vi "2DMain.vi"() -> (0 "Timestep":dbl=0.1 format="%#_13g", 1 "Heading":dbl[](array[numeric]), 2 "Right":cluster{"Distance":dbl[], "Velocity":dbl[]}, 3 "Left":cluster{"Distance":dbl[], "Velocity":dbl[]})   [LabVIEW 2016]
panel:
  out "x-y":dbl
  out "XY Graph":cluster{"X":dbl, "Y":dbl}[](graph)
  in  "TrackWidth":dbl=35.0 format="%#_13g"
  out "Distance":cluster{"Array Out":dbl[], "Array Out":dbl[]}[](graph)=[{"Array Out"=[0.0, 0.1, 0.2, 0.30000000000000004, 0.4, 0.5, 0.6, 0.7, 0.7999999999999999, 0.8999999999999999, 0.9999999999999999, 1.0999999999999999, 1.1999999999999997, 1.2999999999999998, 1.4, 1.5, 1.6, 1.7000000000000002, 1.8000000000000003, 1.9000000000000004, 2.0000000000000004, 2.1000000000000005, 2.2000000000000006, 2.3000000000000007, 2.400000000000001, 2.500000000000001, 2.600000000000001, 2.700000000000001, 2.800000000000001, 2.9000000000000012, 3.0000000000000013, 3.1000000000000014, 3.2000000000000015, 3.3000000000000016, 3.4000000000000017, 3.5000000000000018, 3.600000000000002, 3.700000000000002, 3.800000000000002, 3.900000000000002, 4.000000000000002, 4.100000000000001, 4.200000000000001, 4.300000000000001, 4.4, 4.5, 4.6, 4.699999999999999, 4.799999999999999, 4.899999999999999, 4.999999999999998, 5.099999999999998, 5.1999999999999975, 5.299999999999997, 5.399999999999997, 5.4999999999999964, 5.599999999999996, 5.699999999999996, 5.799999999999995, 5.899999999999995, 5.999999999999995, 6.099999999999994, 6.199999999999994, 6.299999999999994, 6.399999999999993, 6.499999999999993, 6.5999999999999925, 6.699999999999992, 6.799999999999992, 6.8999999999999915, 6.999999999999991, 7.099999999999991, 7.19999999999999, 7.29999999999999, 7.39999999999999, 7.499999999999989], "Array Out"=[0.20069481389041308, 1.2735479131566998, 2.860563643560315, 4.677475723799337, 6.602913279626835, 8.567527988927633, 10.53108018964165, 12.465647282368936, 14.34875346161623, 16.16309622777655, 17.898491074990865, 19.549502803192667, 21.10424300305833, 22.544365069194978, 23.85409275892922, 25.03102772342022, 26.085867448969292, 27.022262629224457, 27.841084013292193, 28.562821763985134, 29.232471840215105, 29.873513699283382, 30.508866157063213, 31.172262554607624, 31.908022069990984, 32.78038389904512, 33.86754429730758, 35.198256581265305, 36.75501986546203, 38.50844318386972, 40.44050862786903, 42.54224982283954, 44.78915116071239, 47.14602178312011, 49.584921471, 52.097800881345535, 54.690898184409775, 57.359640143421814, 60.0931923583142, 62.893846806981905, 65.79097479873057, 68.83230748850526, 72.05193120455107, 75.47740260353666, 79.15300666582458, 83.15137230577258, 87.55638168234262, 92.42537513448103, 97.79978506553392, 103.7283633518359, 110.27176098442025, 117.47770658119887, 125.34310783591802, 133.82920697375735, 142.8898773894898, 152.48590627079324, 162.58103064590355, 173.12865405386947, 184.07735731984107, 195.38107047923268, 207.00308349309873, 218.91193352626502, 231.07343083234156, 243.45198855767703, 256.01410216111213, 268.72824012658504, 281.5595738656088, 294.46074577221134, 307.3634720865251, 320.16447276700615, 332.6976768600146, 344.6827382996951, 355.6340519955303, 364.70338314474, 370.3292731264785, 371.34805932997506]}, {"Array Out"=[0.0, 0.1, 0.2, 0.30000000000000004, 0.4, 0.5, 0.6, 0.7, 0.7999999999999999, 0.8999999999999999, 0.9999999999999999, 1.0999999999999999, 1.1999999999999997, 1.2999999999999998, 1.4, 1.5, 1.6, 1.7000000000000002, 1.8000000000000003, 1.9000000000000004, 2.0000000000000004, 2.1000000000000005, 2.2000000000000006, 2.3000000000000007, 2.400000000000001, 2.500000000000001, 2.600000000000001, 2.700000000000001, 2.800000000000001, 2.9000000000000012, 3.0000000000000013, 3.1000000000000014, 3.2000000000000015, 3.3000000000000016, 3.4000000000000017, 3.5000000000000018, 3.600000000000002, 3.700000000000002, 3.800000000000002, 3.900000000000002, 4.000000000000002, 4.100000000000001, 4.200000000000001, 4.300000000000001, 4.4, 4.5, 4.6, 4.699999999999999, 4.799999999999999, 4.899999999999999, 4.999999999999998, 5.099999999999998, 5.1999999999999975, 5.299999999999997, 5.399999999999997, 5.4999999999999964, 5.599999999999996, 5.699999999999996, 5.799999999999995, 5.899999999999995, 5.999999999999995, 6.099999999999994, 6.199999999999994, 6.299999999999994, 6.399999999999993, 6.499999999999993, 6.5999999999999925, 6.699999999999992, 6.799999999999992, 6.8999999999999915, 6.999999999999991, 7.099999999999991, 7.19999999999999, 7.29999999999999, 7.39999999999999, 7.499999999999989], "Array Out"=[0.2117191306056528, 1.3507882424896287, 3.071429044529173, 5.09397779407175, 7.301900538479339, 9.628251136963636, 12.034681936226827, 14.503404614724442, 17.02963034745262, 19.613660791751258, 22.25469422033156, 24.951328686393314, 27.711896764961377, 30.553446132360143, 33.49237898778358, 36.53443998973933, 39.67669409791384, 42.929661075996734, 46.31492189548162, 49.84503113661403, 53.50368108524415, 57.25169961687586, 61.07026124095799, 64.95859991137544, 68.90728696067245, 72.88101782758629, 76.83587578292126, 80.76784216096199, 84.70462040360079, 88.6778427280159, 92.70471482207125, 96.79005649072815, 100.94903919796458, 105.2061488333065, 109.58233928983002, 114.08475664593064, 118.71116835031577, 123.47309491255056, 128.3941338888642, 133.49475313859787, 138.77995304825606, 144.24552491424538, 149.90687713291584, 155.7961174670011, 161.94399225424323, 168.36714991065222, 175.07505744482475, 182.09686270564254, 189.47668975565475, 197.25604197786453, 205.4591611195571, 214.09006503805574, 223.14687047737073, 232.6258465985691, 242.52047336593304, 252.81806385202069, 263.4961069829394, 274.5251855181033, 285.87506411948084, 297.5184169240899, 309.4300792332615, 321.5837023958519, 333.95091437242615, 346.5036236619891, 359.2151167805168, 372.0578239392519, 384.9981906850866, 397.9905683314788, 410.969322166184, 423.8337224292351, 436.4191499472047, 448.4455434819155, 459.42763327185486, 468.5178463185088, 474.1549337579138, 475.1756544408442]}]
  in  "Path":i32=4
  in  "Timestep":dbl=0.1 format="%#_13g"
  out "Pos":cluster{"Array Out":dbl[], "Array Out":dbl[]}[](graph)=[{"Array Out"=[0.0, 0.0, 100.0, 100.0], "Array Out"=[0.0, -50.0, -50.0, 300.0]}, {"Array Out"=[0.0, 0.23102521238156823, 0.46462967685251366, 0.7037123278438489, 0.9517380195633947, 1.212752350834045, 1.4907899822064303, 1.78783247902104, 2.1065958337168587, 2.451695954720305, 2.8296673375725714, 3.247334487022741, 3.706724316460749, 4.211245916492695, 4.768155922064141, 5.388574268428332, 6.084254547225372, 6.857720318418225, 7.713840686939641, 8.664326744157881, 9.727605490171953, 10.922685952772534, 12.250880804587691, 13.716104501567363, 15.332115456656412, 17.121095424852708, 19.101090310427278, 21.251474961621344, 23.547168687359076, 25.970948218634163, 28.514853498873496, 31.173537193331367, 33.9260087077582, 36.751125048786044, 39.63255921600619, 42.55890760852029, 45.520822161399416, 48.504522369702826, 51.495479207803186, 54.47917940610018, 57.44109393904035, 60.367442301904724, 63.248876430343955, 66.07399272417004, 68.82646418372462, 71.48514781641364, 74.02905302884325, 76.4528324873993, 78.74852613667896, 80.89891070878437, 82.87890551366146, 84.66788540053744, 86.28389627482022, 87.7491198925626, 89.07731466758672, 90.27239505652396, 91.3356737325474, 92.28615972405139, 93.14228003158937, 93.91574574676325, 94.61142597452503, 95.23184427472546, 95.78875423897482, 96.29327580240847, 96.75266559972492, 97.17033272118528, 97.54830407983745, 97.89340418031219, 98.21216751811241, 98.50921000167841, 98.78724762354712, 99.04826194932421, 99.29628764016333, 99.53537029562708, 99.76897477062725, 100.0], "Array Out"=[0.0, -1.827838650398022, -3.65375518167116, -5.475589233211732, -7.290758689387357, -9.096248608842847, -10.889052113698222, -12.66769215834793, -14.430144140207465, -16.1729671902586, -17.89128995963179, -19.58002374541511, -21.237652967227923, -22.86162855610636, -24.446528413729688, -25.98404181136415, -27.46536978319958, -28.888565190622653, -30.249889534074487, -31.540434698254117, -32.74617284968212, -33.85245754230255, -34.85753541640947, -35.75725126468736, -36.5393970689817, -37.18439938874207, -37.674159806617034, -38.017116888370275, -38.221986911053236, -38.28800121444147, -38.20416326811608, -37.95711557222517, -37.55408282907005, -36.998920290461676, -36.28324747689388, -35.386328053162075, -34.28454694169509, -32.97910678617733, -31.4655419732727, -29.722082598161755, -27.70960719661141, -25.385571609721282, -22.745546720347345, -19.776058061619167, -16.436505113053137, -12.659603644587932, -8.375157173488198, -3.5804811976422233, 1.737307919479062, 7.6291113212396535, 14.178887353926195, 21.456950034459567, 29.39106322953373, 37.89510823042944, 46.915601776628804, 56.43664528918128, 66.45254738703716, 76.89163453916119, 87.68459791049352, 98.78739611010738, 110.18168332188421, 121.85794172593427, 133.7721115823067, 145.88252235746378, 158.16198204859364, 170.59771431455354, 183.18212283436563, 195.8896453923813, 208.6958071543085, 221.58331952589336, 234.54200992609125, 247.5644566117797, 260.6355487239612, 273.7401345254334, 286.86523733837987, 300.0]}, {"Array Out"=[17.361870832049785, 17.589538187103535, 17.815857798056786, 18.042596925983897, 18.271683704856557, 18.506023628599557, 18.751734565427235, 19.008441820362023, 19.27328878543838, 19.543098566247437, 19.817797247594193, 20.111683112592367, 20.418804411748653, 20.721624708223516, 20.996721817172322, 21.228727153803682, 21.46022876404934, 21.67174743661132, 21.804621956763874, 21.789771454866482, 21.61567635194309, 21.482648386286343, 21.408110180164382, 21.340039996418675, 21.267603745103752, 21.32315569414887, 21.85726926108888, 22.807010778665354, 24.023623763946112, 25.394524261530325, 26.89571010192149, 28.638122467704868, 30.55162586861914, 32.53275092193286, 34.50431716952587, 36.4576564551441, 38.50617093018464, 40.6028384312195, 42.66652607308066, 44.644190057731024, 46.55766616939471, 48.54539998819105, 50.5701354162769, 52.569682235036375, 54.516392831550185, 56.43771311124984, 58.41118035051687, 60.38605479951565, 62.30924164299841, 64.14759026827126, 65.88476780432264, 67.51996237076557, 69.03800784797089, 70.43579160738425, 71.71356515707643, 72.87017958701705, 73.90776528104465, 74.8409562086548, 75.68459052136886, 76.44827251516784, 77.13607793295802, 77.75093135418209, 78.303920722879, 78.80550946903678, 79.26252745611387, 79.67822071408006, 80.05475373216495, 80.3988230045449, 80.71681410433365, 81.0132366438934, 81.290761777104, 81.55141158543043, 81.79919935740034, 82.03814145672865, 82.27168110629135, 82.5027063356641], "Array Out"=[2.194411358706214, 0.39297816023924836, -1.376721434461866, -3.1063950891235277, -4.786865429183404, -6.414314882292096, -8.006381113569976, -9.553111301648318, -11.030930539782403, -12.413451693458054, -13.689690007205483, -14.90629445979662, -16.04569968462976, -17.0601294262637, -17.897967580376175, -18.544985650268515, -19.108970027110566, -19.57220321067363, -19.872034109856507, -19.96577698641954, -19.903907816382578, -19.897630656856172, -19.94461651489742, -20.005247977157666, -20.076712634852967, -20.196383333498815, -20.392566199778283, -20.58638803608492, -20.7284740974416, -20.797497064426906, -20.77922784039909, -20.641756142831962, -20.38249174219275, -20.014947853899738, -19.551507175517234, -18.984354563260755, -18.2519343004436, -17.36458178743611, -16.355956057541146, -15.247173806826824, -14.005556701122641, -12.482497730495313, -10.683228274119283, -8.645757157642022, -6.363181039259199, -3.725136184586079, -0.48009206903298374, 3.3555590796430605, 7.737301697462016, 12.693029122630946, 18.356121309072584, 24.949618894374467, 32.36248248111438, 40.444355901732294, 49.095097804671475, 58.28404799375175, 68.03937031541905, 78.2754243737801, 88.90077099222853, 99.8538757880656, 111.11023640388856, 122.6750607285158, 134.50053241837068, 146.53676135767063, 158.74940669686964, 171.123088020486, 183.65719781102453, 196.32511006889226, 209.09905512638045, 221.95870767658198, 234.8926992832377, 247.89646164714847, 260.95476906353554, 274.05155539695886, 287.17299442439236, 300.3077570860125]}, {"Array Out"=[-17.361870832049785, -17.1274877623404, -16.88659844435176, -16.6351722702962, -16.36820766572977, -16.080518926931468, -15.770154601014376, -15.432776862319942, -15.06009711800466, -14.639706656806828, -14.158462572449052, -13.617014138546885, -13.005355778827154, -12.299132875238124, -11.460409973044035, -10.45157861694702, -9.291719669598594, -7.9563067997748655, -6.376940582884591, -4.461117966550717, -2.16046537159918, 0.36272351925873103, 3.093651429011002, 6.092169006716055, 9.396627168209074, 12.919035155556548, 16.344911359765675, 19.695939144577338, 23.070713610772042, 26.547372175738, 30.133996895825504, 33.708951918957865, 37.30039154689726, 40.96949917563923, 44.76080126248652, 48.66015876189649, 52.53547339261419, 56.40620630818615, 60.32443234252571, 64.31416875446934, 68.324521708686, 72.1894846156184, 75.92761744441101, 79.57830321330371, 83.13653553589907, 86.53258252157744, 89.64692570716963, 92.51961017528296, 95.18781063035951, 97.65023114929748, 99.8730432230003, 101.81580843030932, 103.52978470166956, 105.06244817774096, 106.44106417809701, 107.67461052603088, 108.76358218405016, 109.73136323944797, 110.59996954180987, 111.38321897835866, 112.08677401609205, 112.71275719526884, 113.27358775507065, 113.78104213578017, 114.24280374333597, 114.6624447282905, 115.04185442750995, 115.38798535607948, 115.70752093189117, 116.00518335946342, 116.28373346999024, 116.545112313218, 116.79337592292632, 117.0325991345255, 117.26626843496315, 117.4972936643359], "Array Out"=[-2.19441135870622, -4.048655461035298, -5.930788928880457, -7.8447833772999385, -9.794651949591312, -11.778182335393597, -13.77172311382647, -15.782273015047544, -17.829357740632524, -19.932482687059153, -22.092889912058098, -24.2537530310336, -26.42960624982609, -28.663127685949025, -30.995089247083204, -33.423097972459786, -35.821769539288596, -38.20492717057168, -40.627744958292475, -43.11509241008869, -45.588437882981665, -47.80728442774894, -49.77045431792152, -51.50925455221706, -53.00208150311043, -54.17241544398533, -54.95575341345578, -55.44784574065564, -55.715499724664866, -55.77850536445604, -55.62909869583308, -55.272475001618375, -54.72567391594734, -53.98289272702361, -53.014987778270516, -51.7883015430634, -50.31715958294657, -48.59363178491856, -46.57512788900425, -44.19699138949669, -41.41365769210018, -38.28864548894725, -34.807865166575404, -30.90635896559631, -26.50982918684707, -21.594071104589787, -16.270222277943414, -10.516521474927508, -4.26268585850389, 2.5651935198483606, 10.001653398779801, 17.964281174544666, 26.419643977953086, 35.34586055912659, 44.73610574858614, 54.58924258461081, 64.86572445865527, 75.50784470454228, 86.46842482875851, 97.72091643214917, 109.25313023987987, 121.04082272335275, 133.04369074624276, 145.22828335725694, 157.57455740031764, 170.0723406086211, 182.70704785770673, 195.45418071587036, 208.29255918223654, 221.20793137520474, 234.1913205689448, 247.2324515764109, 260.3163283843869, 273.42871365390795, 286.5574802523674, 299.6922429139875]}]
  in  "B":dbl=0.3 format="%#_13g"
  in  "A":dbl=0.1 format="%#_13g"
  out "Vel":cluster{"Array Out":dbl[], "Array Out":dbl[]}[](graph)=[{"Array Out"=[0.0, 0.1, 0.2, 0.30000000000000004, 0.4, 0.5, 0.6, 0.7, 0.7999999999999999, 0.8999999999999999, 0.9999999999999999, 1.0999999999999999, 1.1999999999999997, 1.2999999999999998, 1.4, 1.5, 1.6, 1.7000000000000002, 1.8000000000000003, 1.9000000000000004, 2.0000000000000004, 2.1000000000000005, 2.2000000000000006, 2.3000000000000007, 2.400000000000001, 2.500000000000001, 2.600000000000001, 2.700000000000001, 2.800000000000001, 2.9000000000000012, 3.0000000000000013, 3.1000000000000014, 3.2000000000000015, 3.3000000000000016, 3.4000000000000017, 3.5000000000000018, 3.600000000000002, 3.700000000000002, 3.800000000000002, 3.900000000000002, 4.000000000000002, 4.100000000000001, 4.200000000000001, 4.300000000000001, 4.4, 4.5, 4.6, 4.699999999999999, 4.799999999999999, 4.899999999999999, 4.999999999999998, 5.099999999999998, 5.1999999999999975, 5.299999999999997, 5.399999999999997, 5.4999999999999964, 5.599999999999996, 5.699999999999996, 5.799999999999995, 5.899999999999995, 5.999999999999995, 6.099999999999994, 6.199999999999994, 6.299999999999994, 6.399999999999993, 6.499999999999993, 6.5999999999999925, 6.699999999999992, 6.799999999999992, 6.8999999999999915, 6.999999999999991, 7.099999999999991, 7.19999999999999, 7.29999999999999, 7.39999999999999, 7.499999999999989], "Array Out"=[0.0, 12.372404710634475, 16.867961965733866, 19.38524707805461, 20.774503850816224, 21.516879350956227, 21.88575500916673, 22.03750338231366, 22.059246850404637, 21.99898976068586, 21.884595775786014, 21.735465316179884, 21.567838010185906, 21.39086636490795, 21.21078614022004, 21.036380652168358, 20.88260524384004, 20.769595460208766, 20.71554064077986, 20.741238149163674, 20.87312553452902, 21.139138505559412, 21.558196840969877, 22.146332757903, 22.920286281934025, 23.884942406325237, 25.00730511015754, 26.201615050928723, 27.406330399265517, 28.598837650755197, 29.777101396449172, 30.93184938112929, 32.03182897947415, 33.07141598551832, 34.072723255157534, 35.07007214021115, 36.090131871364406, 37.14130978100209, 38.25204996283135, 39.474815512695244, 40.87180169401338, 42.49139031558557, 44.35340950392369, 46.50833340172636, 49.038853444879535, 52.025168577610394, 55.492180787293826, 59.38244543220561, 63.69363759700799, 68.4639215492525, 73.68404574590186, 79.19222262081749, 84.65051888907514, 89.87067775320472, 94.81830414769881, 99.51459563457516, 103.93164470775784, 107.95370522362096, 111.55450817401655, 114.78566877837973, 117.71476648458234, 120.36550738532917, 122.69738889857928, 124.70620834771844, 126.41578314831844, 127.8388568944075, 128.93413980879347, 129.57559553511445, 129.5699618807708, 128.5889586621701, 126.03622897115463, 120.82507088621556, 111.00713371098406, 93.14849572458364, 61.185206037126065, 0.0]}, {"Array Out"=[0.0, 0.1, 0.2, 0.30000000000000004, 0.4, 0.5, 0.6, 0.7, 0.7999999999999999, 0.8999999999999999, 0.9999999999999999, 1.0999999999999999, 1.1999999999999997, 1.2999999999999998, 1.4, 1.5, 1.6, 1.7000000000000002, 1.8000000000000003, 1.9000000000000004, 2.0000000000000004, 2.1000000000000005, 2.2000000000000006, 2.3000000000000007, 2.400000000000001, 2.500000000000001, 2.600000000000001, 2.700000000000001, 2.800000000000001, 2.9000000000000012, 3.0000000000000013, 3.1000000000000014, 3.2000000000000015, 3.3000000000000016, 3.4000000000000017, 3.5000000000000018, 3.600000000000002, 3.700000000000002, 3.800000000000002, 3.900000000000002, 4.000000000000002, 4.100000000000001, 4.200000000000001, 4.300000000000001, 4.4, 4.5, 4.6, 4.699999999999999, 4.799999999999999, 4.899999999999999, 4.999999999999998, 5.099999999999998, 5.1999999999999975, 5.299999999999997, 5.399999999999997, 5.4999999999999964, 5.599999999999996, 5.699999999999996, 5.799999999999995, 5.899999999999995, 5.999999999999995, 6.099999999999994, 6.199999999999994, 6.299999999999994, 6.399999999999993, 6.499999999999993, 6.5999999999999925, 6.699999999999992, 6.799999999999992, 6.8999999999999915, 6.999999999999991, 7.099999999999991, 7.19999999999999, 7.29999999999999, 7.39999999999999, 7.499999999999989], "Array Out"=[0.0, 12.703147836339168, 17.53155536768189, 20.40907881530594, 22.18505434364899, 23.326068474553402, 24.091707667195205, 24.69294881245726, 25.259857792832722, 25.841163979902532, 26.4173129454754, 26.95158995301414, 27.574395206173122, 28.384913936377217, 29.378911092243946, 30.435413020053282, 31.40309694488795, 32.48744569086545, 33.82513897662405, 35.32764757173127, 36.670825204395705, 37.50804852849331, 38.178092579533704, 38.89327859829959, 39.54911325231494, 39.83149135026113, 39.54877336147123, 39.264892523952234, 39.30963922516325, 39.70324513372229, 40.270719704855075, 40.8262016901782, 41.54497365384626, 42.53286612862268, 43.75013995217846, 45.0380014540742, 46.24289559756238, 47.57511841878443, 49.172224461387486, 50.99832231448317, 52.87164126470022, 54.6271072062081, 56.55424186982691, 58.83705843471155, 61.45194443644167, 64.22765105405034, 67.02691073189621, 70.13915806871688, 73.72477264230297, 77.75137436280403, 82.03086323906707, 86.3123211824826, 90.57408714092081, 94.79965661273292, 98.96585368004982, 103.01453470890381, 106.83143664959356, 110.34230654784649, 113.5440492688524, 116.47421245939738, 119.16026917009916, 121.58444941050175, 123.71932294331766, 125.57097741068446, 127.1593247877209, 128.4813105500948, 129.477862536004, 130.02924405597452, 129.94782002362786, 128.90470593182337, 126.29737203214363, 121.03145701777747, 111.160411979395, 93.25228246100522, 61.243240975823106, 0.0]}, {"Array Out"=[0.0, 0.1, 0.2, 0.30000000000000004, 0.4, 0.5, 0.6, 0.7, 0.7999999999999999, 0.8999999999999999, 0.9999999999999999, 1.0999999999999999, 1.1999999999999997, 1.2999999999999998, 1.4, 1.5, 1.6, 1.7000000000000002, 1.8000000000000003, 1.9000000000000004, 2.0000000000000004, 2.1000000000000005, 2.2000000000000006, 2.3000000000000007, 2.400000000000001, 2.500000000000001, 2.600000000000001, 2.700000000000001, 2.800000000000001, 2.9000000000000012, 3.0000000000000013, 3.1000000000000014, 3.2000000000000015, 3.3000000000000016, 3.4000000000000017, 3.5000000000000018, 3.600000000000002, 3.700000000000002, 3.800000000000002, 3.900000000000002, 4.000000000000002, 4.100000000000001, 4.200000000000001, 4.300000000000001, 4.4, 4.5, 4.6, 4.699999999999999, 4.799999999999999, 4.899999999999999, 4.999999999999998, 5.099999999999998, 5.1999999999999975, 5.299999999999997, 5.399999999999997, 5.4999999999999964, 5.599999999999996, 5.699999999999996, 5.799999999999995, 5.899999999999995, 5.999999999999995, 6.099999999999994, 6.199999999999994, 6.299999999999994, 6.399999999999993, 6.499999999999993, 6.5999999999999925, 6.699999999999992, 6.799999999999992, 6.8999999999999915, 6.999999999999991, 7.099999999999991, 7.19999999999999, 7.29999999999999, 7.39999999999999, 7.499999999999989], "Array Out"=[0.0, 12.041688833424784, 16.204430622278075, 18.36153250167981, 19.36416418534402, 19.70806410659394, 19.68046194632811, 19.383220150934577, 18.86068301357076, 18.160418549620026, 17.358208757568306, 16.530437252965662, 15.580745922677252, 14.430991048264993, 13.102613852461802, 11.742214925942376, 10.544624313228791, 9.369671354086913, 8.16040108573351, 7.118007347043244, 6.671834567670051, 6.373658956074809, 6.2960411521273825, 6.563323902205564, 7.254447091715027, 8.564458653936002, 10.829428035789238, 13.34745309865494, 15.623496607054237, 17.56435752493153, 19.324472397681014, 21.061679524302914, 22.53328120333792, 23.619275934716914, 24.40185240225773, 25.107295729045656, 25.941729302291556, 26.711625245642534, 27.336287255860423, 27.95635862445902, 28.87754516636604, 30.3611402149965, 32.15785536012971, 34.18486130723312, 36.630983350072995, 39.827449029750035, 43.96115892780746, 48.62847785322212, 53.664536787609045, 59.17797085951554, 65.33827695244722, 72.07277928575733, 78.72734171124067, 84.941929152429, 90.67088994940376, 96.0147359939041, 101.03189895318627, 105.56513069996929, 109.56498272489092, 113.09713435876397, 116.26926940354987, 119.14656885900025, 121.67545715042685, 123.84144090388503, 125.6722427541605, 127.19640428557923, 128.3904180318958, 129.12194792826241, 129.19210465120622, 128.27321232573897, 125.77508687469972, 120.61868575596885, 110.85385648225208, 93.04471006513418, 61.127172209794075, 0.0]}]
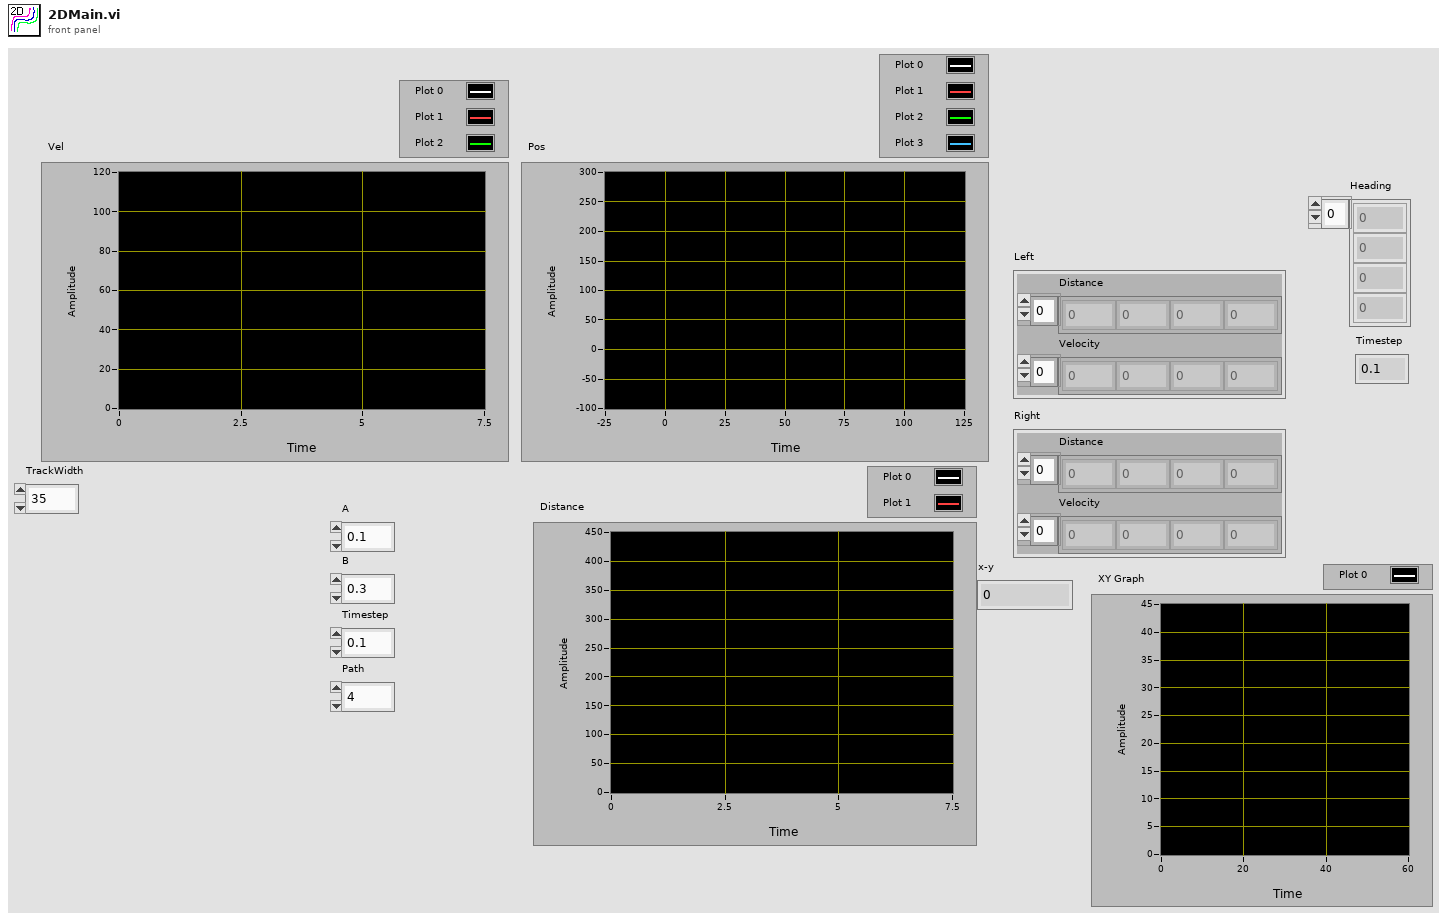
[diagram p1: front panel]
types:
  T1 = cluster{"transposed array":dbl[], "transposed array":dbl[]}
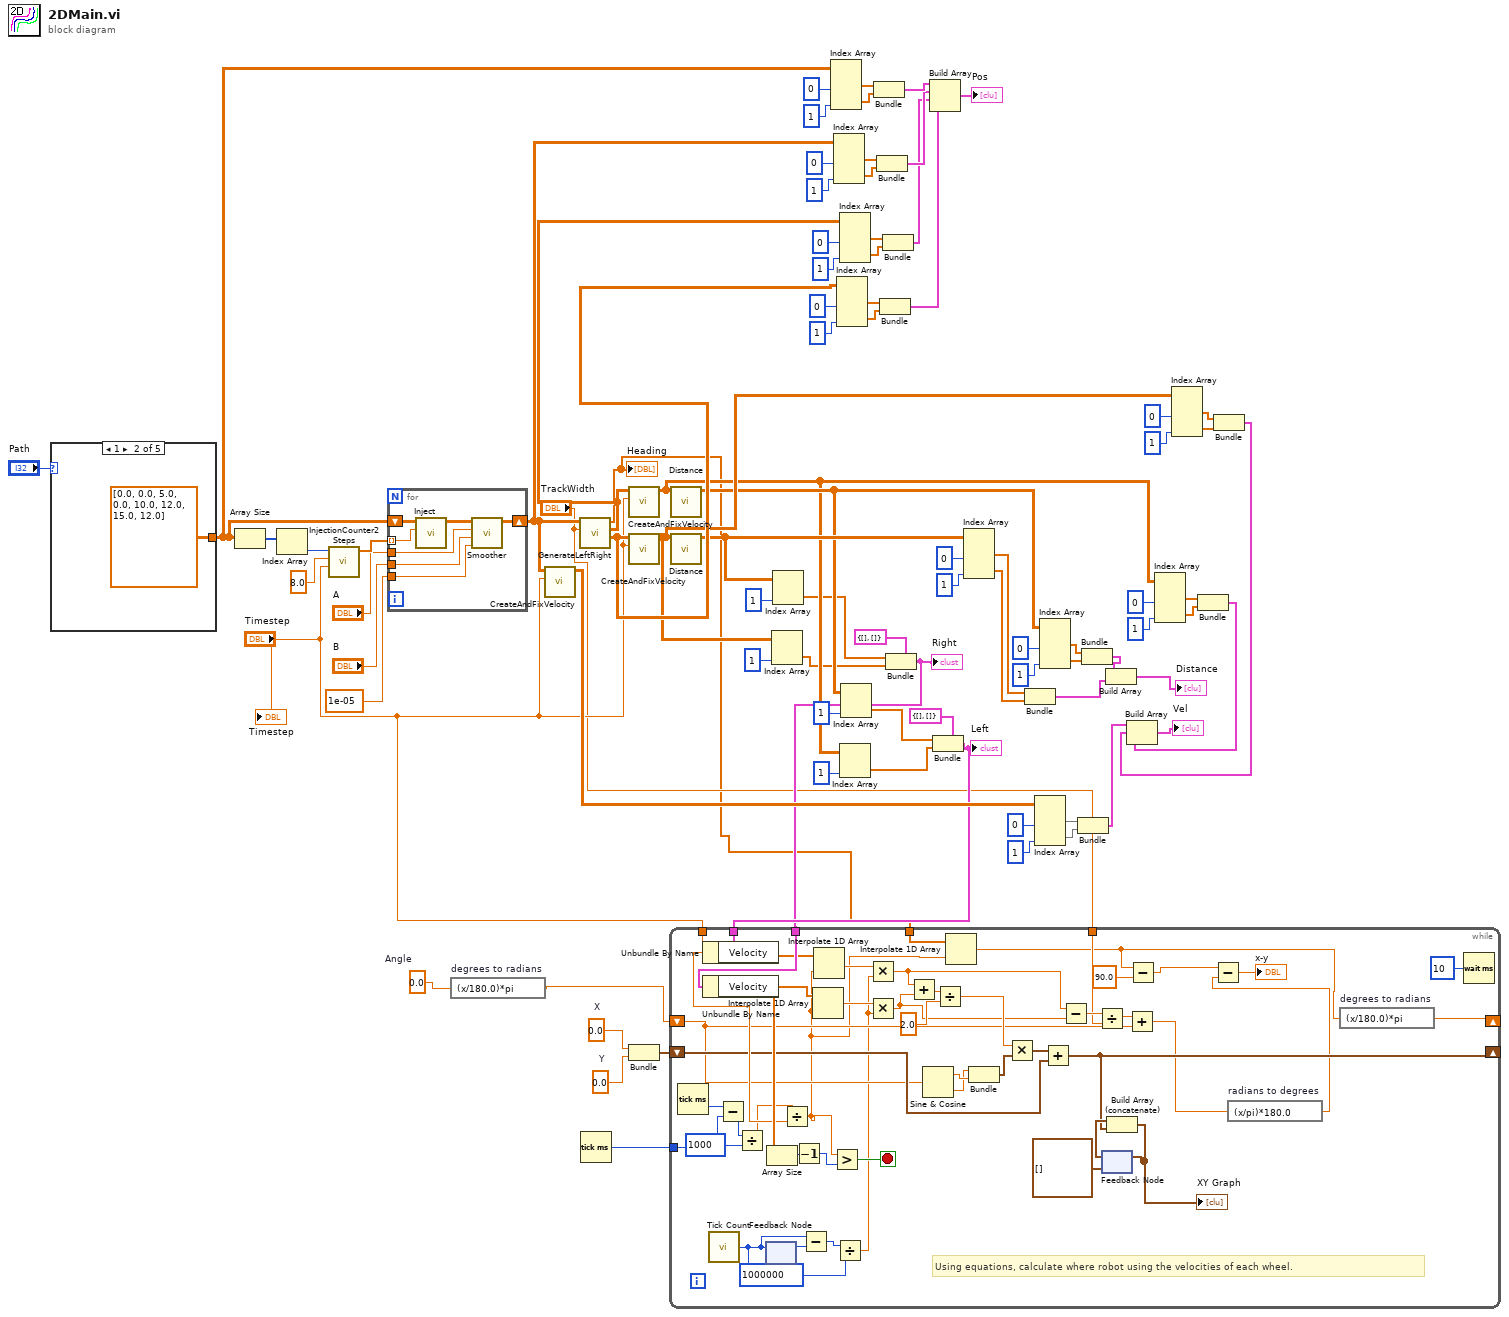
[diagram p0: block diagram]
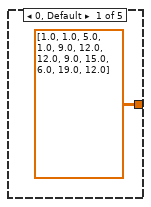
[diagram p2: hidden frame]
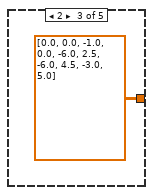
[diagram p3: hidden frame]
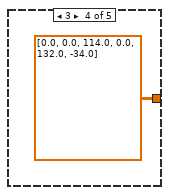
[diagram p4: hidden frame]
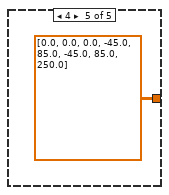
[diagram p5: hidden frame]
diagram:
  w9 = 0.0  # Y
  w8 = 0.0  # X
  w2 = 0.0  # Angle
  n1 = case shown="1" "Path" {
    tunnel: [dbl[][] [[1.0, 1.0], [5.0, 1.0], [9.0, 12.0], [12.0, 9.0], [15.0, 6.0], [19.0, 12.0]] ("transposed array") dbl[][] [[0.0, 0.0], [5.0, 0.0], [10.0, 12.0], [15.0, 12.0]] ("transposed array") dbl[][] [[0.0, 0.0], [-1.0, 0.0], [-6.0, 2.5], [-6.0, 4.5], [-3.0, 5.0]] ("transposed array") dbl[][] [[0.0, 0.0], [114.0, 0.0], [132.0, -34.0]] ("transposed array") dbl[][] [[0.0, 0.0], [0.0, -45.0], [85.0, -45.0], [85.0, 250.0]] ("transposed array")] -> w60
    frame 0, Default {
    }
    frame 1 {
    }
    frame 2 {
    }
    frame 3 {
    }
    frame 4 {
    }
  }
  n2 = Array Size(array=w60) -> (size(s)=w82:i32[])
  n3 = Index Array(array=w82) -> (element=w81:i32)  [unwired: 1 in]
  n4 = call "InjectionCounter2Steps.vi"("Timestep"="Timestep", "Time"=8.0, "NumPoints"=w81) -> ("Array"=w79:dbl[])  [unwired: 8 in]
  n5 = for {
    tunnel: w79 -> [w98] mode=indexing
    shift-right: [w95] -> w40
    shift-left: w60 -> [w97]
    tunnel: "A" -> [w94]
    tunnel: "B" -> [w93]
    tunnel: 1e-05 ("tolerance") -> [w92]
    n6 = call "Inject.vi"("NumToInject"=w98, "Array In"=w97) -> ("Array Out"=w96:dbl[][])  [unwired: 9 in]
    n7 = call "Smoother.vi"("tolerance"=w92, "B"=w93, "A"=w94, "Array In"=w96) -> ("Smooth Array"=w95:dbl[][])  [unwired: 7 in]
  }
  n8 = expression code="(x/180.0)*pi" "degrees to radians"(w2) -> (w1:dbl)
  n9 = call "CreateAndFixVelocity.vi"("Timestep"="Timestep", "Points In"=w40) -> ("Fixed Vel"=w27:dbl[][])  [unwired: 9 in]
  n10 = call "GenerateLeftRight.vi"("TrackWidth"="TrackWidth", "SmoothPath"=w40) -> ("Right"=w41:dbl[][], "Left"=w42:dbl[][], "Heading"=w3:dbl[])  [unwired: 7 in]
  "Heading" <- w3
  n11 = Tick Count (ms)() -> (millisecond timer value=w5:u32)
  n12 = call "CreateAndFixVelocity.vi"("Timestep"="Timestep", "Points In"=w42) -> ("Fixed Vel"=w16:dbl[][])  [unwired: 9 in]
  n13 = call "CreateAndFixVelocity.vi"("Timestep"="Timestep", "Points In"=w41) -> ("Fixed Vel"=w24:dbl[][])  [unwired: 9 in]
  n14 = Bundle("X"=w8, "Y"=w9) -> (w7:cluster{"X":dbl, "Y":dbl})  [unwired: 1 in]
  n15 = call "Distance.vi"("Velocity"=w16) -> ("Distance"=w19:dbl[][])  [unwired: 10 in]
  n16 = call "Distance.vi"("Velocity"=w24) -> ("Distance"=w22:dbl[][])  [unwired: 10 in]
  n17 = Index Array(array=w24, index (col)=1 ("disabled index (col)")) -> (element=w14:dbl[])  [unwired: 1 in]
  n18 = Index Array(array=w22, index (col)=1 ("disabled index (col)")) -> (element=w15:dbl[])  [unwired: 1 in]
  n19 = Index Array(array=w60, index (col) #1=0 ("disabled index (col)"), index (col) #2=1 ("index (col)")) -> (element #1=w61:dbl[], element #2=w64:dbl[])  [unwired: 2 in]
  n20 = Index Array(array=w40, index (col) #1=0 ("disabled index (col)"), index (col) #2=1 ("index (col)")) -> (element #1=w57:dbl[], element #2=w54:dbl[])  [unwired: 2 in]
  n21 = Index Array(array=w41, index (col) #1=0 ("disabled index (col)"), index (col) #2=1 ("index (col)")) -> (element #1=w49:dbl[], element #2=w46:dbl[])  [unwired: 2 in]
  n22 = Index Array(array=w42, index (col) #1=0 ("disabled index (col)"), index (col) #2=1 ("index (col)")) -> (element #1=w50:dbl[], element #2=w52:dbl[])  [unwired: 2 in]
  n23 = Index Array(array=w16, index (col)=1) -> (element=w12:dbl[])  [unwired: 1 in]
  n24 = Index Array(array=w19, index (col)=1 ("disabled index (col)")) -> (element=w13:dbl[])  [unwired: 1 in]
  n25 = Bundle("transposed array"=w61, "transposed array"=w64) -> (w58:T1)  [unwired: 1 in]
  n26 = Bundle("transposed array"=w57, "transposed array"=w54) -> (w53:T1)  [unwired: 1 in]
  n27 = Bundle("Right"=w49, "Right"=w46) -> (w44:cluster{"Right":dbl[], "Right":dbl[]})  [unwired: 1 in]
  n28 = Bundle("Left"=w50, "Left"=w52) -> (w43:cluster{"Left":dbl[], "Left":dbl[]})  [unwired: 1 in]
  n29 = Bundle(cluster=cluster{"Distance":dbl[], "Velocity":dbl[]} {"Distance"=[], "Velocity"=[]}, "Distance"=w15, "Velocity"=w14) -> (w10:cluster{"Distance":dbl[], "Velocity":dbl[]})
  "Right" <- w10
  n30 = Build Array(w58, w53, w43, w44) -> (→"Pos":cluster{"Right":dbl[], "Right":dbl[]}[])
  n31 = Bundle(cluster=cluster{"Distance":dbl[], "Velocity":dbl[]} {"Distance"=[], "Velocity"=[]}, "Distance"=w13, "Velocity"=w12) -> (w11:cluster{"Distance":dbl[], "Velocity":dbl[]})
  "Left" <- w11
  n32 = while {
    tunnel: w11 -> [w146]
    tunnel: w10 -> [w145]
    tunnel: "Timestep" -> [w135]
    tunnel: w5 -> [w136]
    tunnel: "TrackWidth" -> [w116]
    shift-right: [w100] -> _
    shift-left: w1 -> [w114]
    shift-right: [w109] -> _
    shift-left: w7 -> [w120]
    tunnel: w3 -> [w107]
    stop <- w133 stop-if-true
    # "Using equations, calculate where robot using the velocities of each wheel."
    n33 = Tick Count (ms)() -> (millisecond timer value=w137:u32)
    n34 = Unbundle By Name(w146) -> ("Velocity"=w139:dbl[])
    n35 = Unbundle By Name(w145) -> ("Velocity"=w138:dbl[])
    n36 = call "Tick Count"() -> ("Tick Count(uSec)"=w143:u32)
    n37 = Subtract(x=w137, y=w136) -> (x-y=w132:u32)
    n38 = Divide(x=w132, y=u32 1000) -> (x/y=w130:dbl)
    n39 = feedback-in #1(w143) -> ()
    n40 = feedback #1(w143) -> (w144:u32)
    n41 = Array Size(array=w138) -> (size(s)=w134:i32)
    n42 = Divide(x=w130, y=w135) -> (x/y=w106:dbl)
    n43 = Decrement(x=w134) -> (x-1=w129:i32)
    n44 = Subtract(x=w143, y=w144) -> (x-y=w142:u32)
    n45 = Interpolate 1D Array(1:w106, 2:w138) -> (0:w113:dbl)
    n46 = Interpolate 1D Array(1:w106, 2:w139) -> (0:w128:dbl)
    n47 = Greater?(x=w106, y=w129) -> (0:w133:bool)
    n48 = Divide(x=w142, y=u32 1000000) -> (x/y=w112:dbl)
    n49 = Multiply(x=w128, y=w112) -> (x*y=w119:dbl)
    n50 = Multiply(x=w113, y=w112) -> (x*y=w118:dbl)
    n51 = Add(x=w119, y=w118) -> (x+y=w127:dbl)
    n52 = Sine & Cosine(0:w114) -> (1:w125:dbl, 2:w124:dbl)
    n53 = Divide(x=w127, y=2.0) -> (x/y=w122:dbl)
    n54 = Interpolate 1D Array(1:w106, 2:w107) -> (0:w99:dbl)
    n55 = Bundle(w124, w125) -> (w123:cluster{dbl, dbl})  [unwired: 1 in]
    n56 = Multiply(x=w122, y=w123) -> (x*y=w121:cluster{dbl, dbl})
    n57 = Add(x=w121, y=w120) -> (x+y=w109:cluster{dbl, dbl})
    n58 = Subtract(x=w119, y=w118) -> (x-y=w117:dbl)
    n59 = Divide(x=w117, y=w116) -> (x/y=w115:dbl)
    n60 = feedback #2(cluster{dbl, dbl}[] []) -> (w110:cluster{dbl, dbl}[])
    n61 = Build Array (concatenate)(w110, w109) -> (w111:cluster{dbl, dbl}[])
    "XY Graph" <- w111
    n62 = feedback-in #2(w111) -> ()
    n63 = Add(x=w115, y=w114) -> (x+y=w105:dbl)
    n64 = Subtract(x=w99, y=90.0) -> (x-y=w101:dbl)
    n65 = expression code="(x/pi)*180.0" "radians to degrees"(w105) -> (w103:dbl)
    n66 = Subtract(x=w101, y=w103) -> (x-y=→"x-y":dbl)
    n67 = expression code="(x/180.0)*pi" "degrees to radians"(w99) -> (w100:dbl)
    n68 = Wait (ms)(milliseconds to wait=u32 10) -> ()  [unwired: 1 out]
  }
  n69 = Index Array(array=w22, index (col) #1=0 ("disabled index (col)"), index (col) #2=1 ("index (col)")) -> (element #1=w32:dbl[], element #2=w31:dbl[])  [unwired: 2 in]
  n70 = Bundle("Distance"=w32, "Distance"=w31) -> (w30:cluster{"Distance":dbl[], "Distance":dbl[]})  [unwired: 1 in]
  n71 = Index Array(array=w27, index (col) #1=0 ("disabled index (col)"), index (col) #2=1 ("index (col)")) -> (element #1=w84:dbl[], element #2=w83:dbl[])  [unwired: 2 in]
  n72 = Index Array(array=w19, index (col) #1=0 ("disabled index (col)"), index (col) #2=1 ("index (col)")) -> (element #1=w37:dbl[], element #2=w36:dbl[])  [unwired: 2 in]
  n73 = Bundle("Fixed Vel"=w84, "Fixed Vel"=w83) -> (w69:cluster{"Fixed Vel":dbl[], "Fixed Vel":dbl[]})  [unwired: 1 in]
  n74 = Bundle("Distance"=w37, "Distance"=w36) -> (w35:cluster{"Distance":dbl[], "Distance":dbl[]})  [unwired: 1 in]
  n75 = Build Array(w35, w30) -> (→"Distance":cluster{"Distance":dbl[], "Distance":dbl[]}[])
  n76 = Index Array(array=w16, index (col) #1=0 ("disabled index (col)"), index (col) #2=1 ("index (col)")) -> (element #1=w75:dbl[], element #2=w65:dbl[])  [unwired: 2 in]
  n77 = Index Array(array=w24, index (col) #1=0 ("disabled index (col)"), index (col) #2=1 ("index (col)")) -> (element #1=w70:dbl[], element #2=w66:dbl[])  [unwired: 2 in]
  n78 = Bundle("Fixed Vel"=w75, "Fixed Vel"=w65) -> (w68:cluster{"Fixed Vel":dbl[], "Fixed Vel":dbl[]})  [unwired: 1 in]
  n79 = Bundle("Fixed Vel"=w70, "Fixed Vel"=w66) -> (w67:cluster{"Fixed Vel":dbl[], "Fixed Vel":dbl[]})  [unwired: 1 in]
  n80 = Build Array(w69, w67, w68) -> (→"Vel":cluster{"Fixed Vel":dbl[], "Fixed Vel":dbl[]}[])
  "Timestep" <- "Timestep"
